vi "Finish.vi"   [LabVIEW 2018]
doc: "This VI is called during exit. It can be used to close I/O refnums, save collected data, etc."
uses:
  <vilib>/Rock Robotics/WPI/Utilities/WPI_GetSetVariantRefNum.vi
types:
  T1 = typedef "WPI_CompressorDevRef.ctl" = cluster{"DevStatus":errorcluster, "Pneumatics Control Module":u8}
  T2 = typedef "WPI_SolenoidDevRef.ctl" = cluster{"DevStatus":errorcluster, "Pneumatics Control Module":u8, "Forward Solenoid Channel":T3, "Reverse Solenoid Channel":T3}
  T3 = typedef "WPI_SolenoidChannel.ctl" = enum8{"Solenoid 0", "Solenoid 1", "Solenoid 2", "Solenoid 3", "Solenoid 4", "Solenoid 5", "Solenoid 6", "Solenoid 7", "Invalid"}
  T4 = typedef "WPI_JoystickDevRef.ctl" = cluster{"Device":T5}
  T5 = typedef "WPI_JoystickDeviceEnum.ctl" = enum16{"USB 0", "USB 1", "USB 2", "USB 3", "USB 4", "USB 5"}
  T6 = typedef "WPI_EncoderDevRef.ctl" = cluster{"DevStatus":errorcluster, "EncoderIndex":T7, "CounterIndex":T8, "DistancePerCount":dbl, "Decoding Type":T9}
  T7 = typedef "FPGA_EncoderIdx.ctl" = enum8{"Enc 0", "Enc 1", "Enc 2", "Enc 3", "Enc 4", "Enc 5", "Enc 6", "Enc 7", "Invalid"}
  T8 = typedef "FPGA_CounterCtrSystemIndex.ctl" = enum8{"Ctr 0", "Ctr 1", "Ctr 2", "Ctr 3", "Ctr 4", "Ctr 5", "Ctr 6", "Ctr 7", "Invalid"}
  T9 = typedef "WPI_EncoderType.ctl" = enum16{"1x", "2x", "4x"}
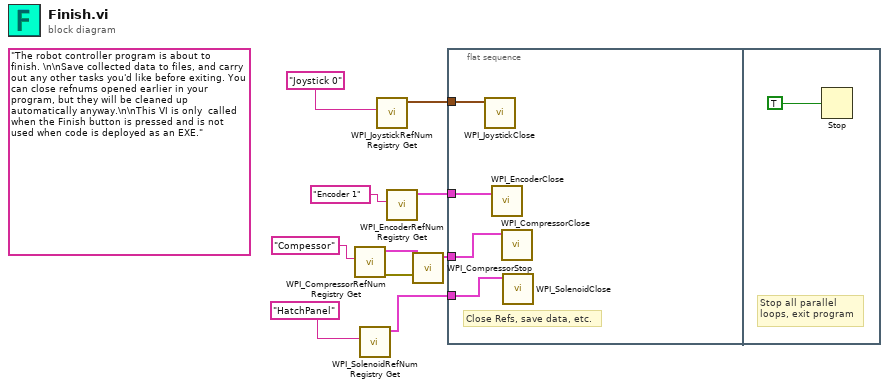
[diagram p0: block diagram]
diagram:
  (unwired) "The robot controller program is about to finish. \n\nSave collected data to files, and carry out any other tasks you'd like before exiting. You can close refnums opened earlier in your program, but they will be cleaned up automatically anyway.\n\nThis VI is only  called when the Finish button is pressed and is not used when code is deployed as an EXE."
  n1 = call <vilib>:"WPI_CompressorRefNum Registry Get.vi"("refnum name"="Compessor") -> ("error out"=w6:errorcluster, "CompressorDevRef"=w5:T1)  [unwired: 9 in]
  n2 = call <vilib>:"WPI_SolenoidRefNum Registry Get.vi"("refnum name"="HatchPanel") -> ("SolenoidDevRef"=w2:T2)  [unwired: 9 in, 1 out]
  n3 = call <vilib>:"WPI_JoystickRefNum Registry Get.vi"("refnum name"="Joystick 0") -> ("JoystickDevRef"=w9:T4)  [unwired: 1 in, 9 out]
  n4 = call <vilib>:"WPI_EncoderRefNum Registry Get.vi"("refnum name"="Encoder 1") -> ("EncoderDevRef"=w7:T6)  [unwired: 9 in, 1 out]
  n5 = call <vilib>:"WPI_CompressorStop.vi"("error in (no error)"=w6, "CompressorDevRef"=w5) -> ("CompressorDevRef"=w1:T1)  [unwired: 8 in, 1 out]
  n6 = flat-sequence {
    tunnel: w9 -> [w14]
    tunnel: w7 -> [w13]
    tunnel: w2 -> [w12]
    tunnel: w1 -> [w11]
    frame #0 {
      # "Close Refs, save data, etc."
      n7 = call <vilib>:"WPI_JoystickClose.vi"("JoystickDevRef"=w14) -> ()  [unwired: 11 out]
      n8 = call <vilib>:"WPI_EncoderClose.vi"("EncoderDevRef"=w13) -> ()  [unwired: 10 in, 1 out]
      n9 = call <vilib>:"WPI_CompressorClose.vi"("CompressorDevRef"=w11) -> ()  [unwired: 10 in, 1 out]
      n10 = call <vilib>:"WPI_SolenoidClose.vi"("SolenoidDevRef"=w12) -> ()  [unwired: 10 in, 1 out]
    }
    frame #1 {
      # "Stop all parallel\nloops, exit program"
      n11 = Stop(stop? (T)=TRUE ("Quit")) -> ()
    }
  }
